vi "Stream-FPGA-)Channel-NoOp.vi"(1 "sentinel in":bool, 5 "valid":bool=TRUE, 7 "channelOp":T1, 9 "size":i32, 11 "element in":T2, 12 "abort in":bool) -> (3 "sentinel out":bool, 6 "wait":refnum<k4>, 10 "count":i32, 13 "retry":bool, 14 "aborted":bool, 15 "element out":T2)   [LabVIEW 2017, in "Stream-t'WPI_EncoderType.ctl'.lvlib"]
doc: "This is a placeholder subVI for the channel's FPGA functionality. The FPGA functionality replaces this subVI when it is installed."
uses:
  <extravilib>/ChannelInstances/Stream-t'WPI_EncoderType.ctl'.lvlib
  <vilib>/Rock Robotics/WPI/Encoder/WPI_EncoderType.ctl
  <extravilib>/ChannelInstances/Stream-t'WPI_EncoderType.ctl'/ChannelOp.ctl
panel:
  in  "probe":bool
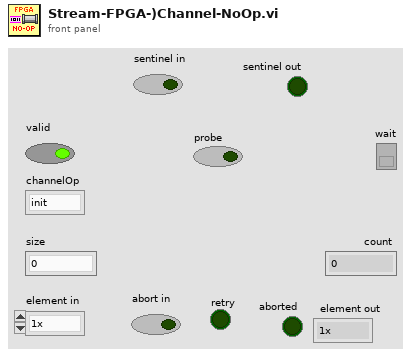
[diagram p1: front panel]
types:
  T1 = typedef "Stream-t'WPI_EncoderType.ctl'.lvlib/ChannelOp.ctl" = enum16{"init", "write", "read", "probe"}
  T2 = typedef "WPI_EncoderType.ctl" = enum16{"1x", "2x", "4x"}
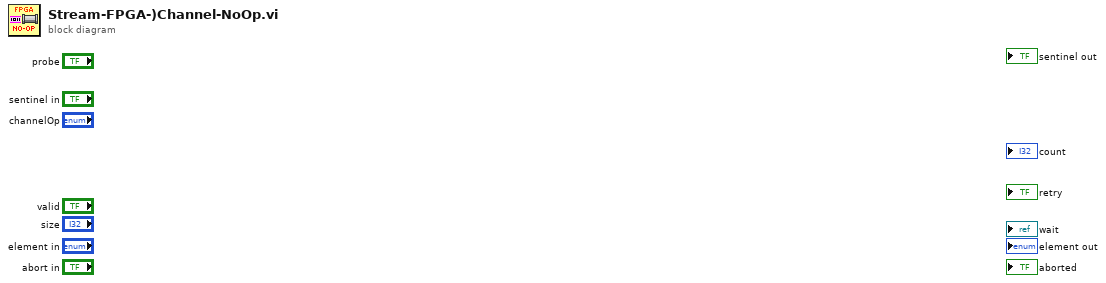
[diagram p0: block diagram]
diagram:
